vi "string2hex.vi"(8 "error in (no error)":errorcluster, 11 "data input":string) -> (0 "error out":errorcluster, 3 "hex display":string)   [LabVIEW 2016]
doc: "Wire anything that is flatten into string to the <b>data input</b>. The VI returns the hex presentation of the <b>data input</b> as well as the line number (#) and ASCII code (separate by \"=>\") via the output terminal <b>hex display</b>."
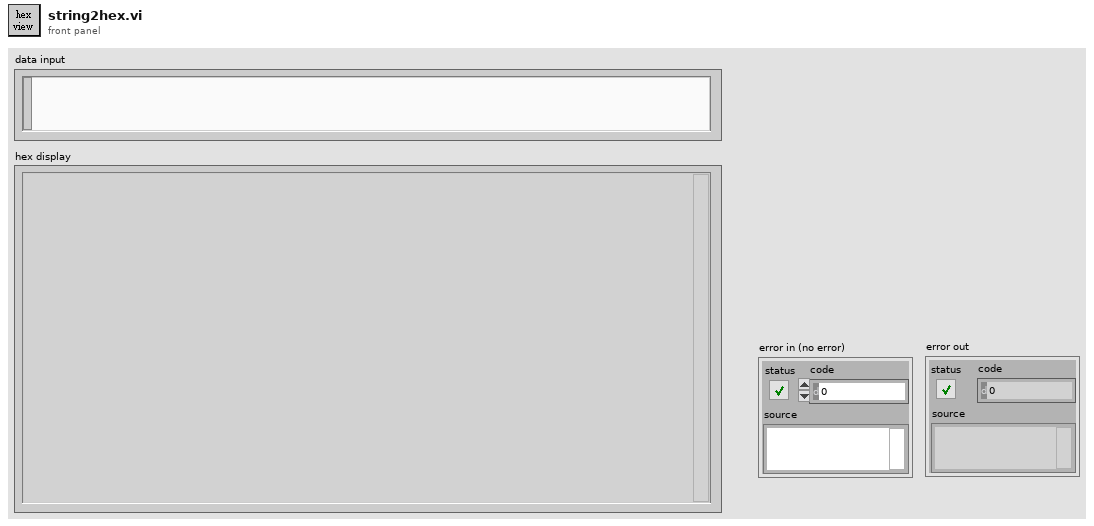
[diagram p1: front panel]
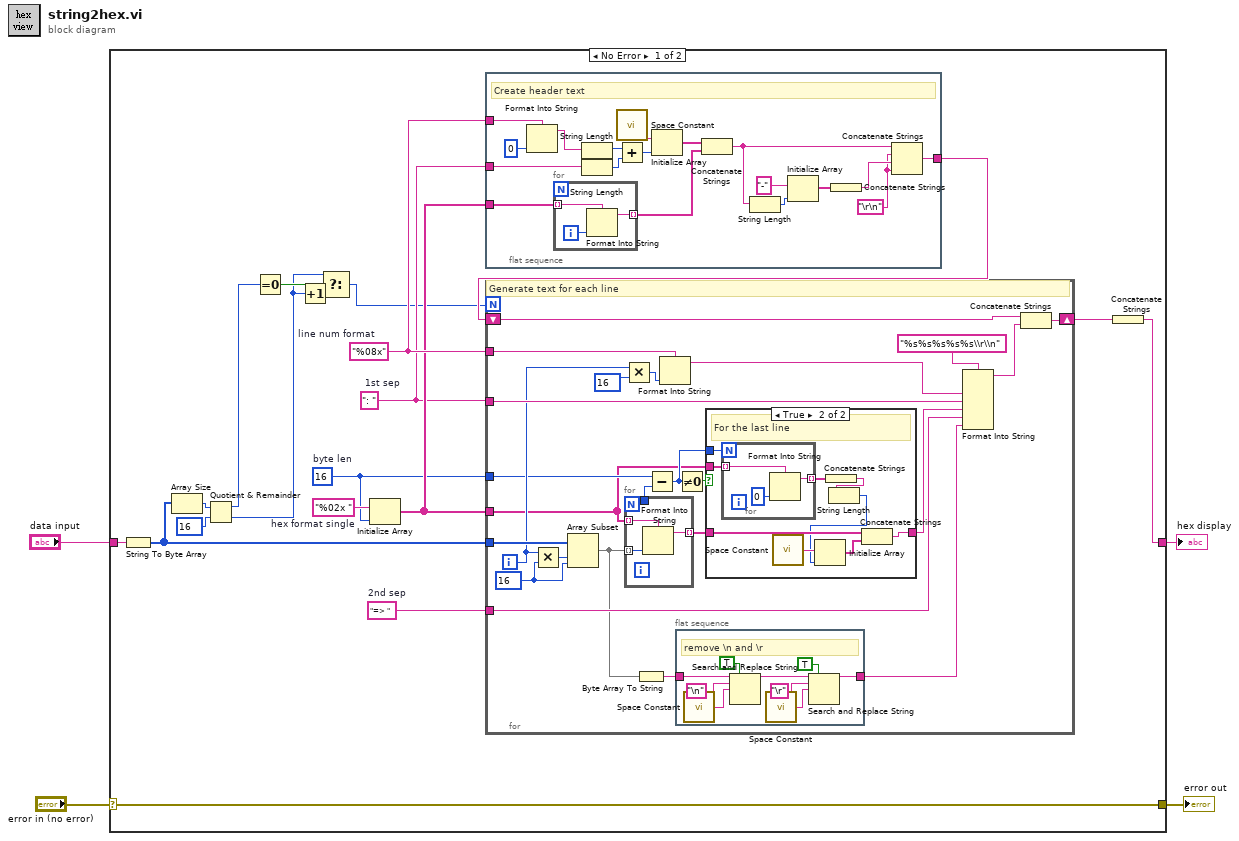
[diagram p0: block diagram]
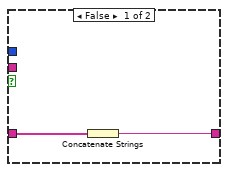
[diagram p2: hidden frame]
diagram:
  n1 = case shown="No Error" "error in (no error)" {
    selector: "error in (no error)" -> [w23 w96]
    tunnel: [w23 w96] -> w3
    tunnel: "data input" -> [w22 _]
    tunnel: [w16 _] -> w1
    frame No Error {
      w18 = "=> "  # 2nd sep
      w10 = 16  # byte len
      w19 = "%02x "  # hex format single
      w13 = ": "  # 1st sep
      w15 = "%08x"  # line num format
      n2 = String To Byte Array(string=w22) -> (unsigned byte array=w11:u8[])
      n3 = Array Size(array=w11) -> (size(s)=w21:i32)
      n4 = Quotient & Remainder(x=w21, y=16) -> (x-y*floor(x/y)=w9:i32, floor(x/y)=w7:i32)
      n5 = Equal To 0?(x=w9) -> (x = 0?=w8:bool)
      n6 = Increment(x=w7) -> (x+1=w5:i32)
      n7 = Select(t=w7, s=w8, f=w5) -> (s? t:f=w6:i32)
      n8 = Initialize Array(w19, w10) -> (w14:string[])
      n9 = flat-sequence {
        tunnel: [w38] -> w12
        tunnel: w15 -> [w25]
        tunnel: w14 -> [w41]
        tunnel: w13 -> [w40]
        frame #0 {
          w33 = "\r\n"
          # "Create header text"
          n10 = Format Into String(format string=w25, 0 ("input 1")) -> (resulting string=w26:string)  [unwired: 2 in, 1 out]
          n11 = for {
            tunnel: w41 -> [w43] mode=indexing
            tunnel: [w42] -> w28 mode=indexing
            i -> [w44]
            n12 = Format Into String(format string=w43, w44) -> (resulting string=w42:string)  [unwired: 2 in, 1 out]
          }
          n13 = String Length(string=w26) -> (length=w32:i32)
          n14 = String Length(string=w40) -> (length=w31:i32)
          n15 = call <vilib>:"Space Constant.vi"() -> ("String"=w39:string)
          n16 = Add(x=w32, y=w31) -> (x+y=w30:i32)
          n17 = Initialize Array(w39, w30) -> (w29:string[])
          n18 = Concatenate Strings(w29, w28) -> (w27:string)
          n19 = String Length(string=w27) -> (length=w37:i32)
          n20 = Initialize Array("-", w37) -> (w35:string[])
          n21 = Concatenate Strings(w35) -> (w34:string)
          n22 = Concatenate Strings(w27, w33, w34, w33) -> (w38:string)
        }
      }
      n23 = for {
        N: w6 -> [_]
        tunnel: w11 -> [w68]
        shift-right: [w67] -> w17
        shift-left: w12 -> [w66]
        tunnel: w15 -> [w60]
        tunnel: w13 -> [w59]
        tunnel: w14 -> [w46]
        tunnel: w18 -> [w58]
        tunnel: w10 -> [w49]
        i -> [w56]
        w55 = 16
        # "Generate text for each line"
        n24 = Multiply(x=w56, y=w55) -> (x*y=w54:i32)
        n25 = Array Subset(array=w68, index=w54, length=w55) -> (w57:u8[])
        n26 = Multiply(x=w56, y=16) -> (x*y=w62:i32)
        n27 = for {
          N -> [w93]
          tunnel: w57 -> [w95] mode=indexing
          tunnel: w46 -> [w92] mode=indexing
          tunnel: [w94] -> w51 mode=indexing
          tunnel: [w93] -> w48
          n28 = Format Into String(format string=w92, w95) -> (resulting string=w94:string)  [unwired: 2 in, 1 out]
        }
        n29 = Byte Array To String(unsigned byte array=w57) -> (string=w53:string)
        n30 = Subtract(x=w49, y=w48) -> (x-y=w47:i32)
        n31 = Format Into String(format string=w60, w62) -> (resulting string=w61:string)  [unwired: 2 in, 1 out]
        n32 = flat-sequence {
          tunnel: w53 -> [w91]
          tunnel: [w83] -> w52
          frame #0 {
            # "remove \\n and \\r"
            n33 = call <vilib>:"Space Constant.vi"() -> ("String"=w88:string)
            n34 = Search and Replace String(replace all?=TRUE ("replace all? (F)"), input string=w91, search string="\n", replace string=w88) -> (result string=w84:string)  [unwired: 4 in, 3 out]
            n35 = call <vilib>:"Space Constant.vi"() -> ("String"=w85:string)
            n36 = Search and Replace String(replace all?=TRUE ("replace all? (F)"), input string=w84, search string="\r", replace string=w85) -> (result string=w83:string)  [unwired: 4 in, 3 out]
          }
        }
        n37 = Not Equal To 0?(x=w47) -> (x != 0?=w45:bool)
        n38 = case shown="True" w45 {
          tunnel: w51 -> [w70 w79]
          tunnel: [w69 w78] -> w50
          tunnel: w47 -> [_ w77]
          tunnel: w46 -> [_ w76]
          frame False {
            n39 = Concatenate Strings(w70) -> (w69:string)
          }
          frame True {
            # "For the last line"
            n40 = for {
              N: w77 -> [_]
              tunnel: w76 -> [w81] mode=indexing
              tunnel: [w80] -> w75 mode=indexing
              n41 = Format Into String(format string=w81, 0 ("input 1")) -> (resulting string=w80:string)  [unwired: 2 in, 1 out]
            }
            n42 = call <vilib>:"Space Constant.vi"() -> ("String"=w73:string)
            n43 = Concatenate Strings(w75) -> (w74:string)
            n44 = String Length(string=w74) -> (length=w72:i32)
            n45 = Initialize Array(w73, w72) -> (w71:string[])
            n46 = Concatenate Strings(w79, w71) -> (w78:string)
          }
        }
        n47 = Format Into String(format string="%s%s%s%s%s\\r\\n", w61, w59, w50, w58, w52) -> (resulting string=w64:string)  [unwired: 2 in, 1 out]
        n48 = Concatenate Strings(w66, w64) -> (w67:string)
      }
      n49 = Concatenate Strings(w17) -> (w16:string)
    }
    frame Error {
    }
  }
  "hex display" <- w1
  "error out" <- w3
